vi "Repeat Message.vi"(4 "First Immediate (F)":bool, 6 "Period ms":u32, 7 "High Priority (F)":bool, 8 "error in (no error)":errorcluster, 9 "Data":variant, 10 "ID":string, 11 "MessageQ in":refnum<class "MessageQ.lvclass">) -> (0 "error out":errorcluster, 2 "Repeat Message Control":refnum<class "Repeat Message Control.lvclass">, 3 "MessageQ out":refnum<class "MessageQ.lvclass">)   [LabVIEW 2020, in "Volatus.lvlib" / "MessageQ.lvclass"]
uses:
  MessageQ.lvclass
  Repeat Message Control/Repeat Message Control.lvclass
  Repeat Message Async.vi
  MessageQ.lvclass/MessageQ.ctl
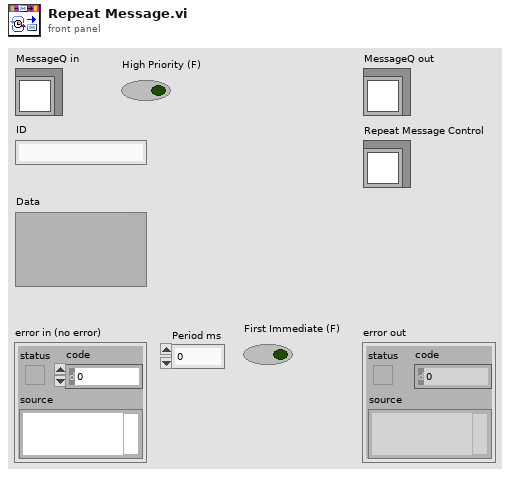
[diagram p1: front panel]
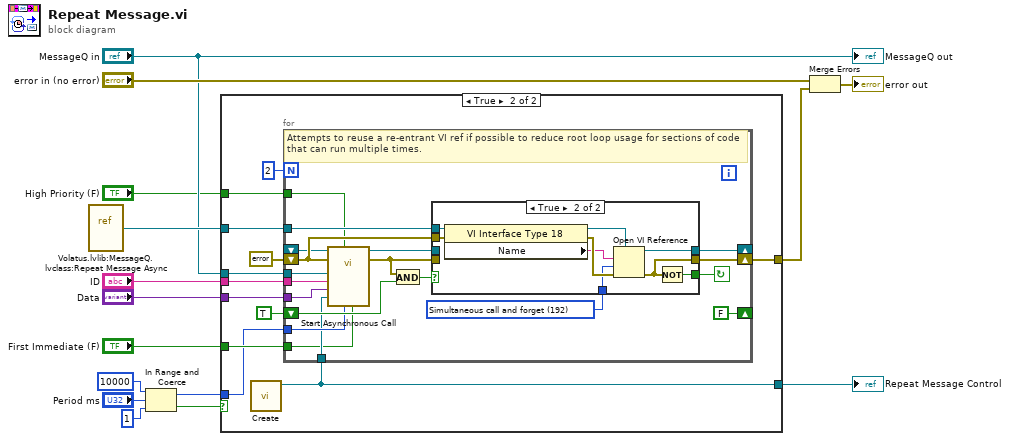
[diagram p0: block diagram]
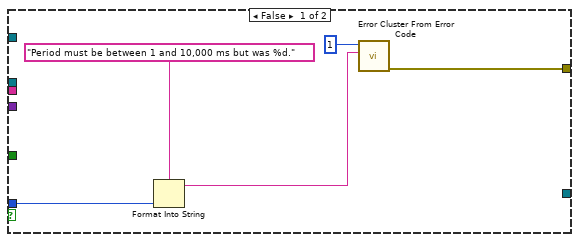
[diagram p2: hidden frame]
diagram:
  n1 = vi-ref "Volatus.lvlib:MessageQ.lvclass:Repeat Message Async.vi"() -> (w14:refnum<vi>)
  n2 = In Range and Coerce(upper limit=u32 10000, x="Period ms", lower limit=u32 1) -> (coerced(x)=w1:u32, In Range?=w2:bool)
  n3 = case shown="True" w2 {
    tunnel: w14 -> [_ w30]
    tunnel: "First Immediate (F)" -> [_ w28]
    tunnel: "Data" -> [_ w27]
    tunnel: "MessageQ in" -> [_ w26]
    tunnel: "ID" -> [_ w25]
    tunnel: "High Priority (F)" -> [_ w24]
    tunnel: [w19 w23] -> w7
    tunnel: [_ w22] -> w6
    tunnel: w1 -> [w17 w21]
    frame False {
      n4 = Format Into String(format string="Period must be between 1 and 10,000 ms but was %d." ("error message (\"\")"), w17) -> (resulting string=w16:string)  [unwired: 2 in, 1 out]
      n5 = call <vilib>:"Error Cluster From Error Code.vi"("error message (\"\")"=w16, "error code (0)"=1) -> ("error out"=w19:errorcluster)  [unwired: 7 in]
    }
    frame True {
      n6 = call "Create.vi"() -> ("Repeat Message Control out"=w22:refnum<class "Repeat Message Control.lvclass">)  [unwired: 10 in, 1 out]
      n7 = for {
        N: 2 -> [_]
        tunnel: w30 -> [w50]
        shift-right: [w49] -> _
        shift-left: _ -> [w48]
        shift-right: [w46] -> w23
        shift-left: errorcluster {"status"=FALSE, "code"=0, "source"=""} ("error constant") -> [w51]
        shift-right: [FALSE] -> _
        shift-left: TRUE -> [w43]
        tunnel: w21 -> [w39]
        tunnel: w28 -> [w33]
        tunnel: w27 -> [w38]
        tunnel: w26 -> [w37]
        tunnel: w25 -> [w36]
        tunnel: w24 -> [w35]
        tunnel: w22 -> [w34]
        stop <- w42 continue-if-true
        w40 = 192 items=["Record modifications"=1, "Open templates for editing"=2, "Prompt user to save"=4, "Prepare for reentrant run"=8, "Prompt to find missing subVIs"=16, "Hide loading dialog box"=32, "Enable simultaneous calls"=64, "Prepare to call and forget"=128, "Simultaneous call and forget"=192, "Prepare to call and collect"=256, "Simultaneous call and collect"=320]
        # "Attempts to reuse a re-entrant VI ref if possible to reduce root loop usage for sections of code that can run multiple times."
        n8 = call-by-ref "Start Asynchronous Call"(reference=w48, error in=w51, "First Immediate (F)"=w33, "Period ms"=w39, "High Priority (F)"=w35, "Repeat Message Control"=w34, "Data"=w38, "ID"=w36, "MessageQ in"=w37) -> (reference out=w47:refnum<vi>, error out=w45:errorcluster)  [unwired: 5 in]
        n9 = And(x=w45, y=w43) -> (x .and. y?=w44:bool)
        n10 = case shown="True" w44 {
          tunnel: w50 -> [_ w61]
          tunnel: w40 -> [_ w59]
          tunnel: [w53 w57] -> w49
          tunnel: w47 -> [w53 _]
          tunnel: [w52 w55] -> w46
          tunnel: w45 -> [w52 _]
          tunnel: w51 -> [_ w56]
          tunnel: [_ w54] -> w42
          frame False {
          }
          frame True {
            n11 = property class="VI Interface Type 18"(reference=w61, error in=w56) -> (reference out=w58:refnum<vi>, error out=w62:errorcluster, "Name"=w60:string)
            n12 = Open VI Reference(type specifier VI Refnum (for type only)=w58, vi path=w60, options=w59, error in (no error)=w62) -> (vi reference=w57:refnum<vi>, error out=w55:errorcluster)  [unwired: 2 in]
            n13 = Not(x=w55) -> (.not. x?=w54:bool)
          }
        }
      }
    }
  }
  "Repeat Message Control" <- w6
  n14 = Merge Errors("error in (no error)", w7) -> (→"error out":errorcluster)
  "MessageQ out" <- "MessageQ in"
